vi "Test Assert Not Equal.vi"(8 "error in (no error)":errorcluster) -> (0 "error out":errorcluster)   [LabVIEW 2009]
uses:
  classes/Assert/Assert.lvclass
  classes/Test/Test.lvclass
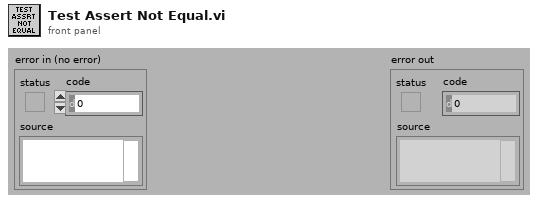
[diagram p1: front panel]
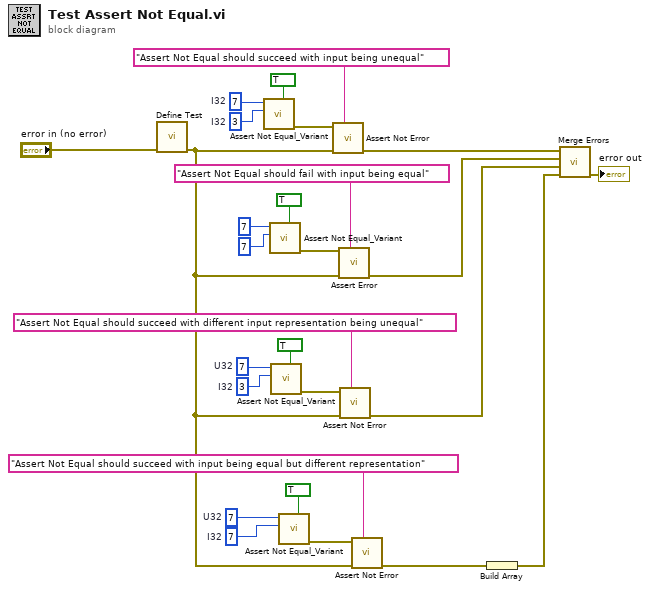
[diagram p0: block diagram]
diagram:
  w6 = 7  # I32
  w7 = u32 7  # U32
  w14 = 3  # I32
  w13 = u32 7  # U32
  w17 = 3  # I32
  w18 = 7  # I32
  n1 = call "Define Test.vi"("error in (no error)"="error in (no error)") -> ("error out"=w3:errorcluster)  [unwired: 10 in]
  n2 = call "Assert Not Equal_Variant.vi"("Assert Only? (F)"=TRUE, "Y"=w17, "X"=w18) -> ("error out"=w28:errorcluster)  [unwired: 8 in]
  n3 = call "Assert Not Equal_Variant.vi"("Assert Only? (F)"=TRUE, "Y"=7, "X"=7) -> ("error out"=w26:errorcluster)  [unwired: 8 in]
  n4 = call "Assert Not Equal_Variant.vi"("Assert Only? (F)"=TRUE, "Y"=w14, "X"=w13) -> ("error out"=w10:errorcluster)  [unwired: 8 in]
  n5 = call "Assert Not Equal_Variant.vi"("Assert Only? (F)"=TRUE, "Y"=w6, "X"=w7) -> ("error out"=w4:errorcluster)  [unwired: 8 in]
  n6 = call "Assert Not Error.vi"("Label"="Assert Not Equal should succeed with input being unequal", "error in (no error)"=w3, "Not Error?"=w28) -> ("error out"=w20:errorcluster)  [unwired: 8 in]
  n7 = call "Assert Error.vi"("Label"="Assert Not Equal should fail with input being equal", "error in (no error)"=w3, "Error?"=w26) -> ("error out"=w21:errorcluster)  [unwired: 8 in]
  n8 = call "Assert Not Error.vi"("Label"="Assert Not Equal should succeed with different input representation being unequal", "error in (no error)"=w3, "Not Error?"=w10) -> ("error out"=w9:errorcluster)  [unwired: 8 in]
  n9 = call "Assert Not Error.vi"("Label"="Assert Not Equal should succeed with input being equal but different representation", "error in (no error)"=w3, "Not Error?"=w4) -> ("error out"=w1:errorcluster)  [unwired: 8 in]
  n10 = Build Array(w1) -> (w5:errorcluster[])
  n11 = call <vilib>:"Merge Errors.vi"("error array in"=w5, "error in 3 (no error)"=w9, "error in 2 (no error)"=w21, "error in 1 (no error)"=w20) -> ("error out"=→"error out":errorcluster)  [unwired: 3 in]
